vi "CANFrameFD_Avg_Length.vi"(0 "Payload Size (bytes)":i32, 1 "Extended ID?":bool) -> (5 "Avg.ArbitrationLength (bits)":i32, 6 "Avg.DataLength (bits)":i32)   [LabVIEW 2019, in "XNET-Bus-Load-Calculator.lvlib" / "CANBus_Load_Calculator.lvclass"]
uses:
  CANBus_Load_Calculator.lvclass
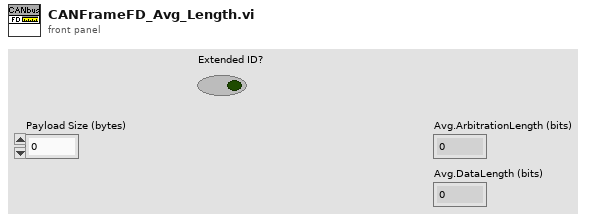
[diagram p1: front panel]
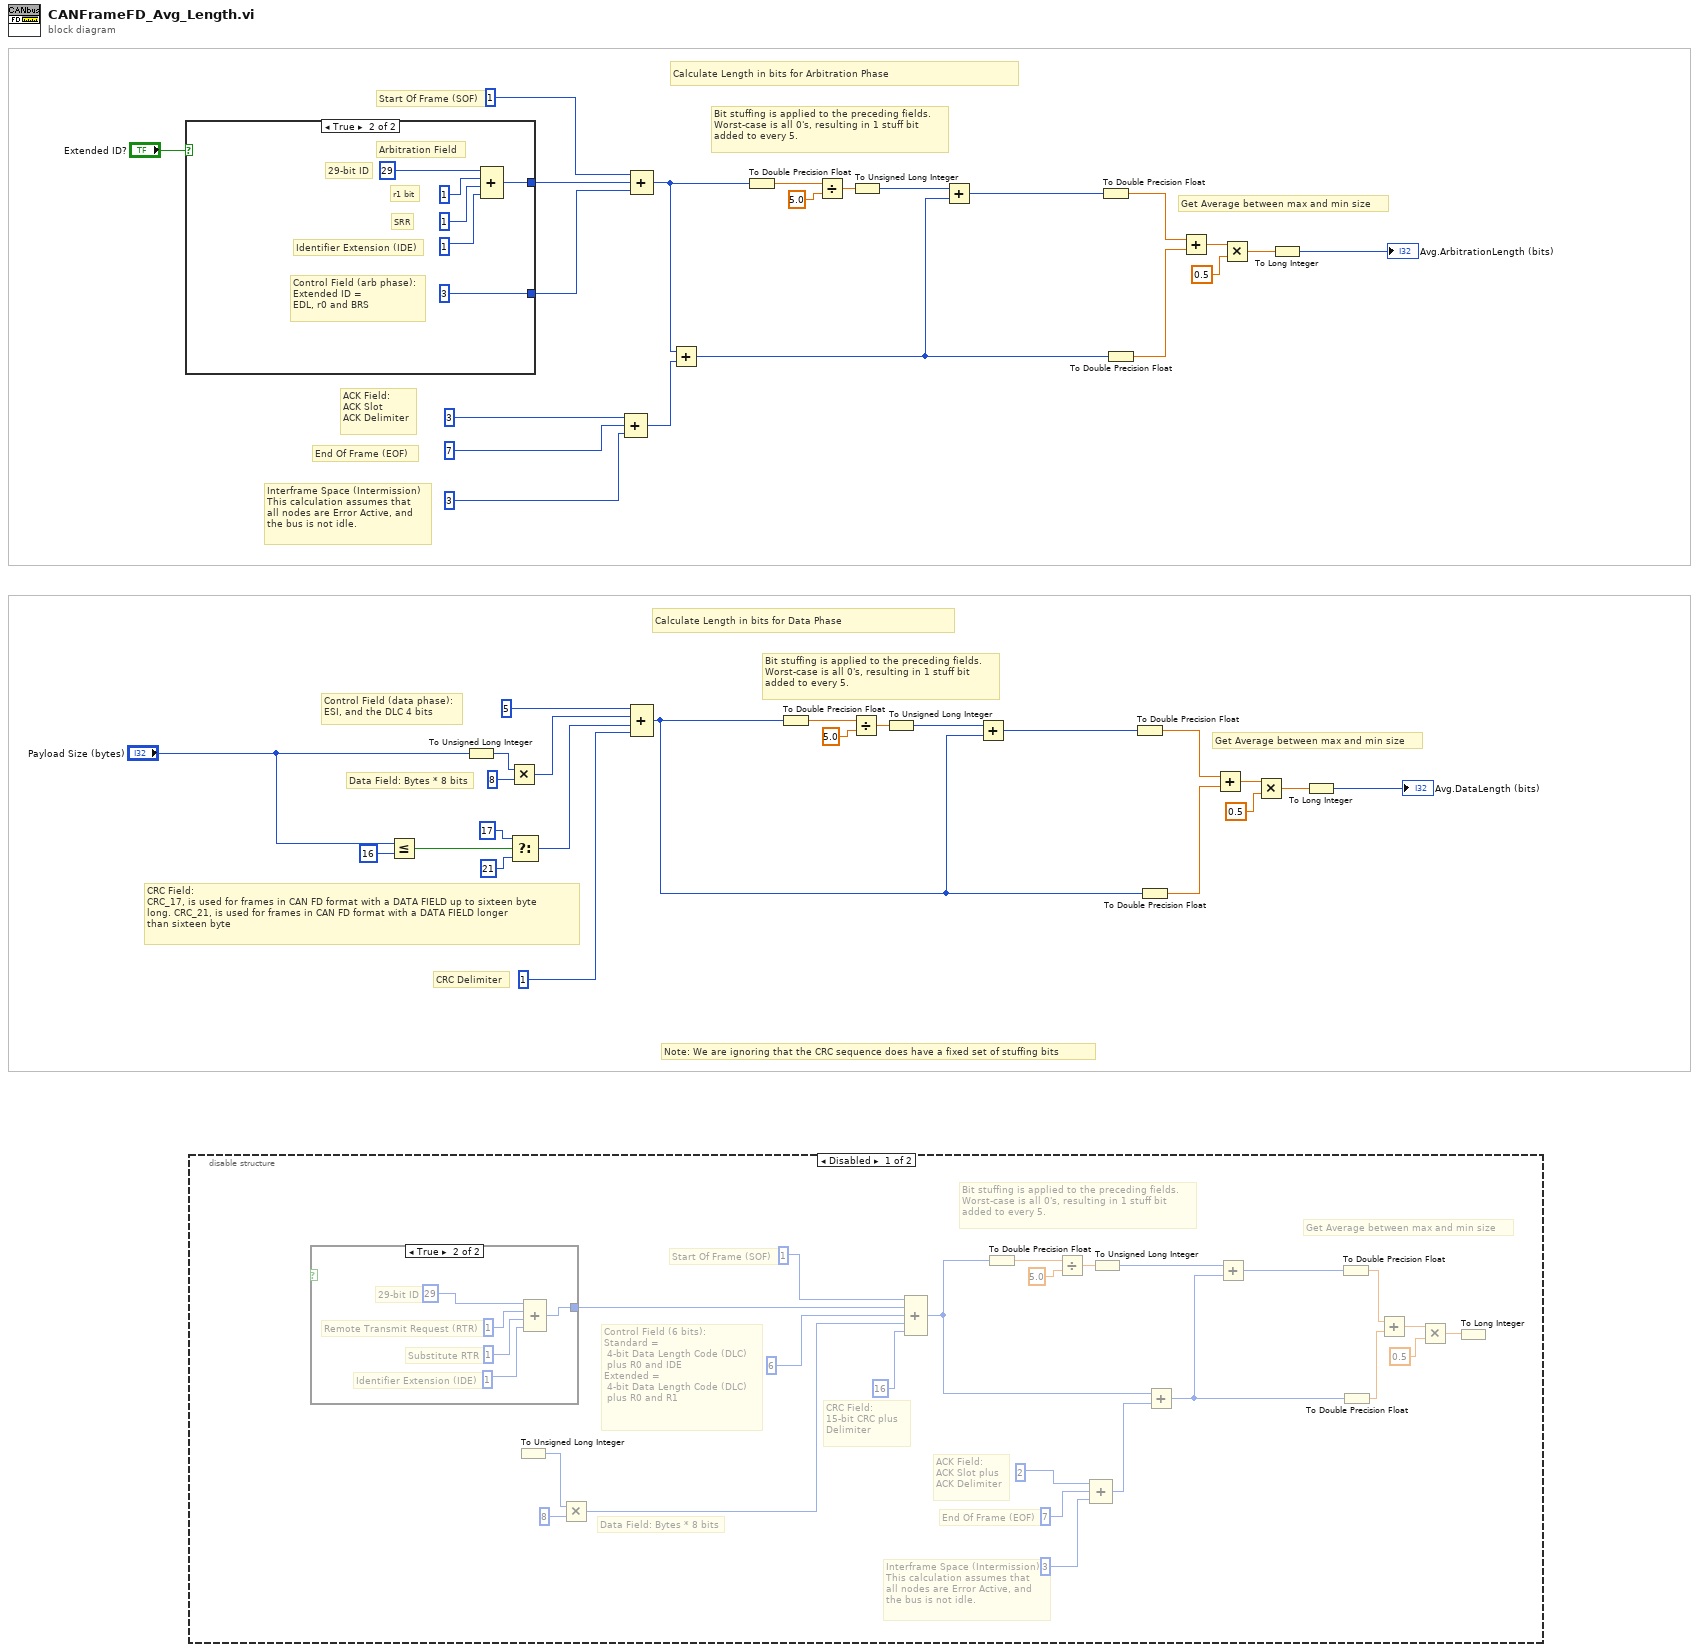
[diagram p0: block diagram]
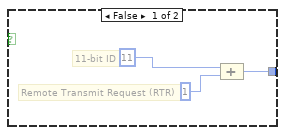
[diagram p2: hidden frame]
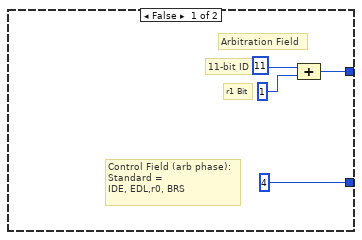
[diagram p4: hidden frame]
diagram:
  # "Note: We are ignoring that the CRC sequence does have a fixed set of stuffing bits"
  # "Get Average between max and min size"
  # "Bit stuffing is applied to the preceding fields.\nWorst-case is all 0's, resulting in 1 stuff bit\nadded to every 5."
  # "Get Average between max and min size"
  # "Bit stuffing is applied to the preceding fields.\nWorst-case is all 0's, resulting in 1 stuff bit\nadded to every 5."
  # "CRC Delimiter"
  # "Calculate Length in bits for Data Phase"
  # "Calculate Length in bits for Arbitration Phase"
  # "Control Field (data phase):\nESI, and the DLC 4 bits"
  # "Interframe Space (Intermission)\nThis calculation assumes that\nall nodes are Error Active, and\nthe bus is not idle."
  # "End Of Frame (EOF)"
  # "ACK Field:\nACK Slot\nACK Delimiter"
  # "CRC Field:\nCRC_17, is used for frames in CAN FD format with a DATA FIELD up to sixteen byte\nlong. CRC_21, is used for frames in CAN FD format with a DATA FIELD longer\nthan sixteen byte"
  # "Data Field: Bytes * 8 bits"
  # "Start Of Frame (SOF)"
  n1 = case shown="True" "Extended ID?" {
    tunnel: [w46 w52] -> w40
    tunnel: [u32 4 u32 3] -> w39
    frame False {
      # "Arbitration Field"
      # "Control Field (arb phase):\nStandard = \nIDE, EDL,r0, BRS"
      # "r1 Bit"
      # "11-bit ID"
      n2 = Compound Arithmetic op=unknown(u32 11, u32 1) -> (w46:u32)
    }
    frame True {
      # "Arbitration Field"
      # "Control Field (arb phase):\nExtended ID = \nEDL, r0 and BRS"
      # "Identifier Extension (IDE)"
      # "SRR"
      # "r1 bit"
      # "29-bit ID"
      n3 = Compound Arithmetic op=unknown(u32 29, u32 1, u32 1, u32 1) -> (w52:u32)
    }
  }
  n4 = disable-structure shown="Disabled" {
    frame Disabled {
      # "Get Average between max and min size"
      # "Interframe Space (Intermission)\nThis calculation assumes that\nall nodes are Error Active, and\nthe bus is not idle."
      # "End Of Frame (EOF)"
      # "ACK Field:\nACK Slot plus\nACK Delimiter"
      # "Bit stuffing is applied to the preceding fields.\nWorst-case is all 0's, resulting in 1 stuff bit\nadded to every 5."
      # "CRC Field:\n15-bit CRC plus \nDelimiter"
      # "Data Field: Bytes * 8 bits"
      # "Control Field (6 bits):\nStandard = \n 4-bit Data Length Code (DLC)\n plus R0 and IDE\nExtended = \n 4-bit Data Length Code (DLC)\n plus R0 and R1"
      # "Start Of Frame (SOF)"
      n5 = case shown="True" w79 {
        tunnel: [w80 w85] -> w78
        frame False {
          # "Remote Transmit Request (RTR)"
          # "11-bit ID"
          n6 = Compound Arithmetic op=ADD(u32 11, u32 1) -> (w80:u32)
        }
        frame True {
          # "Identifier Extension (IDE)"
          # "Substitute RTR"
          # "Remote Transmit Request (RTR)"
          # "29-bit ID"
          n7 = Compound Arithmetic op=unknown(u32 29, u32 1, u32 1, u32 1) -> (w85:u32)
        }
      }
      n8 = To Unsigned Long Integer() -> (number=w68:u32, unsigned 32bit integer=w69:u32)
      n9 = Multiply(x=w69, y=u32 8) -> (x*y=w58:u32)
      n10 = Compound Arithmetic op=ADD(u32 1, w78, u32 6, w58, u32 16) -> (w63:u32)
      n11 = To Double Precision Float(number=w63) -> (double precision float=w70:dbl)
      n12 = Divide(x=w70, y=5.0) -> (x/y=w65:dbl)
      n13 = Compound Arithmetic op=unknown(u32 2, u32 7, u32 3) -> (w64:u32)
      n14 = To Unsigned Long Integer(number=w65) -> (unsigned 32bit integer=w66:u32)
      n15 = Add(x=w63, y=w64) -> (x+y=w72:u32)
      n16 = Add(x=w66, y=w72) -> (x+y=w71:u32)
      n17 = To Double Precision Float(number=w71) -> (double precision float=w73:dbl)
      n18 = To Double Precision Float(number=w72) -> (double precision float=w74:dbl)
      n19 = Add(x=w73, y=w74) -> (x+y=w75:dbl)
      n20 = Multiply(x=w75, y=0.5) -> (x*y=w77:dbl)
      n21 = To Long Integer(number=w77) -> ()  [unwired: 1 out]
    }
    frame Enabled {
    }
  }
  n22 = Less Or Equal?(x="Payload Size (bytes)", y=16) -> (x <= y?=w34:bool)
  n23 = To Unsigned Long Integer(number="Payload Size (bytes)") -> (unsigned 32bit integer=w43:u32)
  n24 = Multiply(x=w43, y=u32 8) -> (x*y=w37:u32)
  n25 = Select(t=u32 17, s=w34, f=u32 21) -> (s? t:f=w31:u32)
  n26 = Compound Arithmetic op=unknown(u32 3, u32 7, u32 3) -> (w26:u32)
  n27 = Compound Arithmetic op=ADD(u32 1, w40, w39) -> (w17:u32)
  n28 = Compound Arithmetic op=ADD(u32 5, w37, w31, u32 1) -> (w2:u32)
  n29 = Add(x=w17, y=w26) -> (x+y=w16:u32)
  n30 = To Double Precision Float(number=w17) -> (double precision float=w22:dbl)
  n31 = To Double Precision Float(number=w2) -> (double precision float=w9:dbl)
  n32 = Divide(x=w22, y=5.0) -> (x/y=w24:dbl)
  n33 = Divide(x=w9, y=5.0) -> (x/y=w11:dbl)
  n34 = To Unsigned Long Integer(number=w24) -> (unsigned 32bit integer=w23:u32)
  n35 = To Unsigned Long Integer(number=w11) -> (unsigned 32bit integer=w10:u32)
  n36 = Add(x=w23, y=w16) -> (x+y=w21:u32)
  n37 = Add(x=w10, y=w2) -> (x+y=w8:u32)
  n38 = To Double Precision Float(number=w21) -> (double precision float=w18:dbl)
  n39 = To Double Precision Float(number=w16) -> (double precision float=w15:dbl)
  n40 = To Double Precision Float(number=w8) -> (double precision float=w5:dbl)
  n41 = To Double Precision Float(number=w2) -> (double precision float=w4:dbl)
  n42 = Add(x=w18, y=w15) -> (x+y=w20:dbl)
  n43 = Add(x=w5, y=w4) -> (x+y=w7:dbl)
  n44 = Multiply(x=w20, y=0.5) -> (x*y=w14:dbl)
  n45 = Multiply(x=w7, y=0.5) -> (x*y=w3:dbl)
  n46 = To Long Integer(number=w14) -> (32bit integer=→"Avg.ArbitrationLength (bits)":i32)
  n47 = To Long Integer(number=w3) -> (32bit integer=→"Avg.DataLength (bits)":i32)
